vi "AuMT8852B Change Register Query.vi"(8 "error in (no error)":errorcluster, 11 "VISA session":refnum<visa-resource-name>) -> (0 "error out":errorcluster, 2 "error code":i32, 3 "VISA session out":refnum<visa-resource-name>, 4 "Flags":T1, 6 "Value":i32)   [LabVIEW 2017]
doc: "Anritsu MT8852B Bluetooth Tester\n\nReturns the current state of the Change Register (CHG) displaying the state of SCO connection, USB status change and AFH status change.\n\nOUTPUTS\nFlags - value of each status message contained in the register.\nStatus - integer value (0-255) of the register; in general, 0 means no error or event to report."
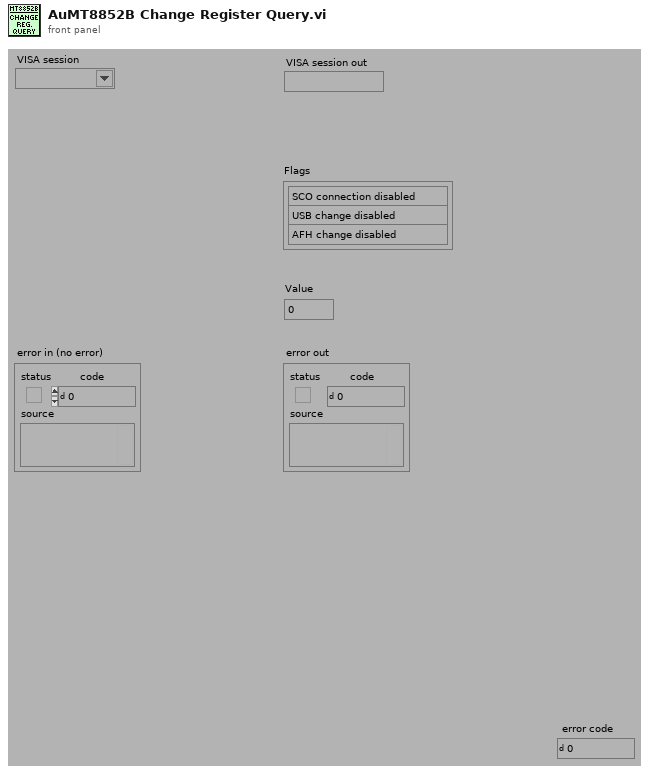
[diagram p1: front panel]
types:
  T1 = cluster{"SCO Connection":enum16{"SCO connection disabled", "SCO connection enabled"}, "USB Change":enum16{"USB change disabled", "USB change enabled"}, "AFH Change":enum16{"AFH change disabled", "AFH change enabled"}}
  T2 = enum16{"Simulate", "Range check", "Cache", "Query instrument status"}
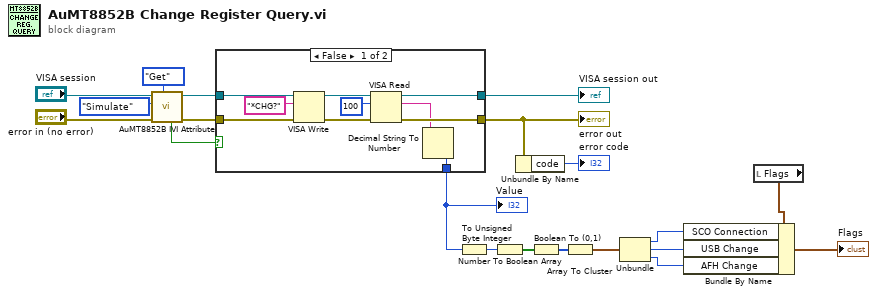
[diagram p0: block diagram]
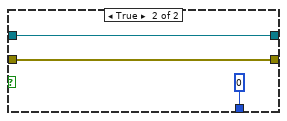
[diagram p2: hidden frame]
diagram:
  n1 = call <instrlib>:"AuMT8852B IVI Attribute.vi"("Set/Get (Set)"=enum16{"Set", "Get"}."Get", "error in (no error)"="error in (no error)", "Flag (Simulate)"=T2."Simulate", "VISA session"="VISA session") -> ("error out"=w16:errorcluster, "VISA session out"=w17:refnum<visa-resource-name>, "Value out"=w13:bool)  [unwired: 5 in]
  n2 = case shown="False" w13 {
    tunnel: [w24 w32] -> w6
    tunnel: [w25 w33] -> w18
    tunnel: w17 -> [w30 w33]
    tunnel: w16 -> [w29 w32]
    tunnel: [w21 0] -> w12
    frame False {
      n3 = VISA Write(VISA resource name=w30, write buffer="*CHG?" ("write buffer (\"\")"), error in (no error)=w29) -> (VISA resource name out=w27:refnum<visa-resource-name>, error out=w26:errorcluster)  [unwired: 1 out]
      n4 = VISA Read(VISA resource name=w27, byte count=u32 100 ("byte count (0)"), error in (no error)=w26) -> (VISA resource name out=w25:refnum<visa-resource-name>, read buffer=w22:string, error out=w24:errorcluster)  [unwired: 1 out]
      n5 = Decimal String To Number(string=w22) -> (number=w21:i32)  [unwired: 2 in, 1 out]
    }
    frame True {
    }
  }
  "error out" <- w6
  "VISA session out" <- w18
  "Value" <- w12
  n6 = To Unsigned Byte Integer(number=w12) -> (unsigned 8bit integer=w11:u8)
  n7 = Number To Boolean Array(number=w11) -> (Boolean array=w10:bool[])
  n8 = Unbundle By Name(w6) -> ("code"=→"error code":i32)
  n9 = Boolean To (0,1)(Boolean=w10) -> (0, 1=w9:i16[])
  n10 = Array To Cluster(array=w9) -> (cluster=w8:cluster{"[0]":i16, "[1]":i16, "[2]":i16})
  n11 = Unbundle(w8) -> ("[0]"=w2:i16, "[1]"=w3:i16, "[2]"=w1:i16)
  n12 = local read "Flags"() -> (w4:T1)
  n13 = Bundle By Name(cluster=w4, "SCO Connection"=w2, "USB Change"=w3, "AFH Change"=w1) -> (→"Flags":T1)
